vi "PEAK_Can_Write.vi"(3 "CAN handle":T1, 7 "MSG type":enum8{"STD", "RTR", "XTD", "XTD RTR", "STATUS"}(ring), 8 "errin":errorcluster, 9 "CAN Data":u8[](array[numeric]) format="%x", 10 "DLC (8)":u8=8, 11 "Identifier":u32=1921 format="%x") -> (0 "errout":errorcluster)   [LabVIEW 2020, in "PEAK_lib_ALEX.lvlib"]
uses:
  PEAK_lib_ALEX.lvlib
  <vilib>/Sylvain.lib/user.lib/PCAN Basic/Controls/Channel.ctl
  <userlib>/PCAN Basic/Controls/CAN MSG Cluster.ctl
  <userlib>/PCAN Basic/PCANBasic.lvlib
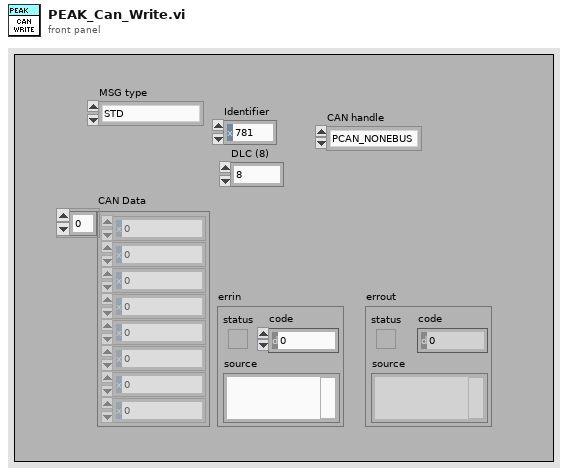
[diagram p1: front panel]
types:
  T1 = typedef "PCANBasic.lvlib/Channel.ctl" = enum16{"PCAN_NONEBUS", "not used1", "not used2", "not used3", "not used4", "not used5", "not used6", "not used7", "not used8", "not used9", "not used10", "not used11", "not used12", "not used13", "not used14", "not used15", "not used16", "not used17", "not used18", "not used19", "not used20", "not used21", "not used22", "not used23", "not used24", "not used25", "not used26", "not used27", "not used28", "not used29", "not used30", "not used31", "not used32", "PCAN_ISABUS1", "PCAN_ISABUS2", "PCAN_ISABUS3", "PCAN_ISABUS4", "PCAN_ISABUS5", "PCAN_ISABUS6", "PCAN_ISABUS7", "PCAN_ISABUS8", "not used41", "not used42", "not used43", "not used44", "not used45", "not used46", "not used47", "not used48", "PCAN_DNGBUS1", "not used50", "not used51", "not used52", "not used53", "not used54", "not used55", "not used56", "not used57", "not used58", "not used59", "not used60", "not used61", "not used62", "not used63", "not used64", "PCAN_PCIBUS1", "PCAN_PCIBUS2", "PCAN_PCIBUS3", "PCAN_PCIBUS4", "PCAN_PCIBUS5", "PCAN_PCIBUS6", "PCAN_PCIBUS7", "PCAN_PCIBUS8", "not used73", "not used74", "not used75", "not used76", "not used77", "not used78", "not used79", "not used80", "PCAN_USBBUS1", "PCAN_USBBUS2", "PCAN_USBBUS3", "PCAN_USBBUS4", "PCAN_USBBUS5", "PCAN_USBBUS6", "PCAN_USBBUS7", "PCAN_USBBUS8", "Not used89", "Not used90", "Not used91", "Not used92", "Not used93", "Not used94", "Not used95", "Not used96", "PCAN_PCCBUS1", "PCAN_PCCBUS2"}
  T2 = typedef "PCANBasic.lvlib/CAN MSG Cluster.ctl" = cluster{"ID":u32, "MSG type":enum8{"STD", "RTR", "XTD", "XTD RTR", "STATUS"}, "LEN":i8, "DATA":u8[]}
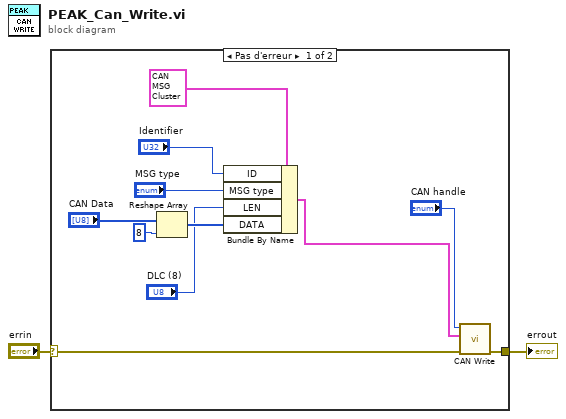
[diagram p0: block diagram]
diagram:
  n1 = case shown="Pas d'erreur" "errin" {
    selector: "errin" -> [w4 w14]
    tunnel: [w10 w14] -> w1
    frame No Error {
      n2 = Reshape Array("CAN Data", 8 ("taille de la dimension")) -> (w8:u8[])
      n3 = Bundle By Name(cluster=T2 {"ID"=0, "MSG type"=enum."STD", "LEN"=0, "DATA"=[0, 0, 0, 0, 0, 0, 0, 0]} ("CAN_Message"), "ID"="Identifier", "MSG type"="MSG type", "LEN"="DLC (8)", "DATA"=w8) -> (w12:T2)
      n4 = call <userlib>:"CAN Write.vi"("error in (no error)"=w4, "CAN_Message"=w12, "Channel"="CAN handle") -> ("error out"=w10:errorcluster)  [unwired: 7 in, 1 out]
    }
    frame Error {
    }
  }
  "errout" <- w1
